vi "Router - Latency Bmk - Serial CVT FGV.vi"() -> ()   [LabVIEW 2016]
uses:
  <vilib>/Utility/error.llb/DialogType.ctl
  <vilib>/NI/Current Value Table/Type Defs/File Format.ctl
  <vilib>/NI/Current Value Table/Type Defs/Single Tag.ctl
  <vilib>/NI/Current Value Table/Type Defs/Data Types.ctl
  <vilib>/NI/Current Value Table/Type Defs/Tag Grouping set.ctl
  <vilib>/pximc/Initialize Reader Session (DBL).vi
  <vilib>/pximc/Initialize Writer Session (DBL).vi
  <vilib>/pximc/Connect (DBL).vi
  <vilib>/pximc/Read (DBL).vi
  <vilib>/pximc/Write (DBL).vi
  <vilib>/pximc/nipximc.lvlib
  <vilib>/NI/Current Value Table/Current Value Table.lvlib
panel:
  in  "Stop Button":bool
  in  "Node 2 Reader Interface":tag="PXI1Slot2" caption="interface"
  in  "Node 2 Reader Connection ID":u16=4
  in  "Node 2 Writer Interface":tag="PXI1Slot2" caption="interface"
  in  "Node 2 Writer Connection ID":u16=3
  in  "Node 1 Reader Interface":tag="PXI1Slot2" caption="interface"
  in  "Node 1 Reader Connection ID":u16=2
  in  "Node 1 Writer Interface":tag="PXI1Slot2" caption="interface"
  in  "Buffer Size":u64=250000 caption="buffer size"
  in  "Connection Timeout (s)":dbl=60.0 caption="timeout in seconds (-1)"
  in  "Node 1 Writer Connection ID":u16=1
  # "Node 1"
  # "Node 2"
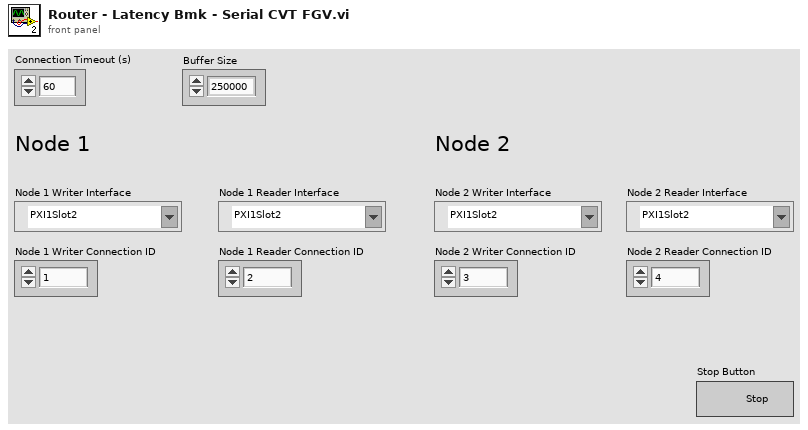
[diagram p1: front panel]
types:
  T1 = typedef "Current Value Table.lvlib/File Format.ctl" = cluster{"Tags":T2[], "Group Listings":T4[]}
  T2 = typedef "Current Value Table.lvlib/Single Tag.ctl" = cluster{"Data Type":T3, "Name":string, "Value":string, "Description":string}
  T3 = typedef "Current Value Table.lvlib/Data Types.ctl" = enum16{"Double", "Single", "I64", "I32", "I16", "I8", "U64", "U32", "U16", "U8", "String", "Boolean", "Array of U8", "Array of U16", "Array of U32", "Array of U64", "Array of I64", "Array of I32", "Array of I16", "Array of I8", "Array of Double", "Array of Single", "Array of Boolean", "Array of String"}
  T4 = typedef "Current Value Table.lvlib/Tag Grouping set.ctl" = cluster{"Group":string, "Tag Names":string[]}
  T5 = typedef "DialogType.ctl" = u16
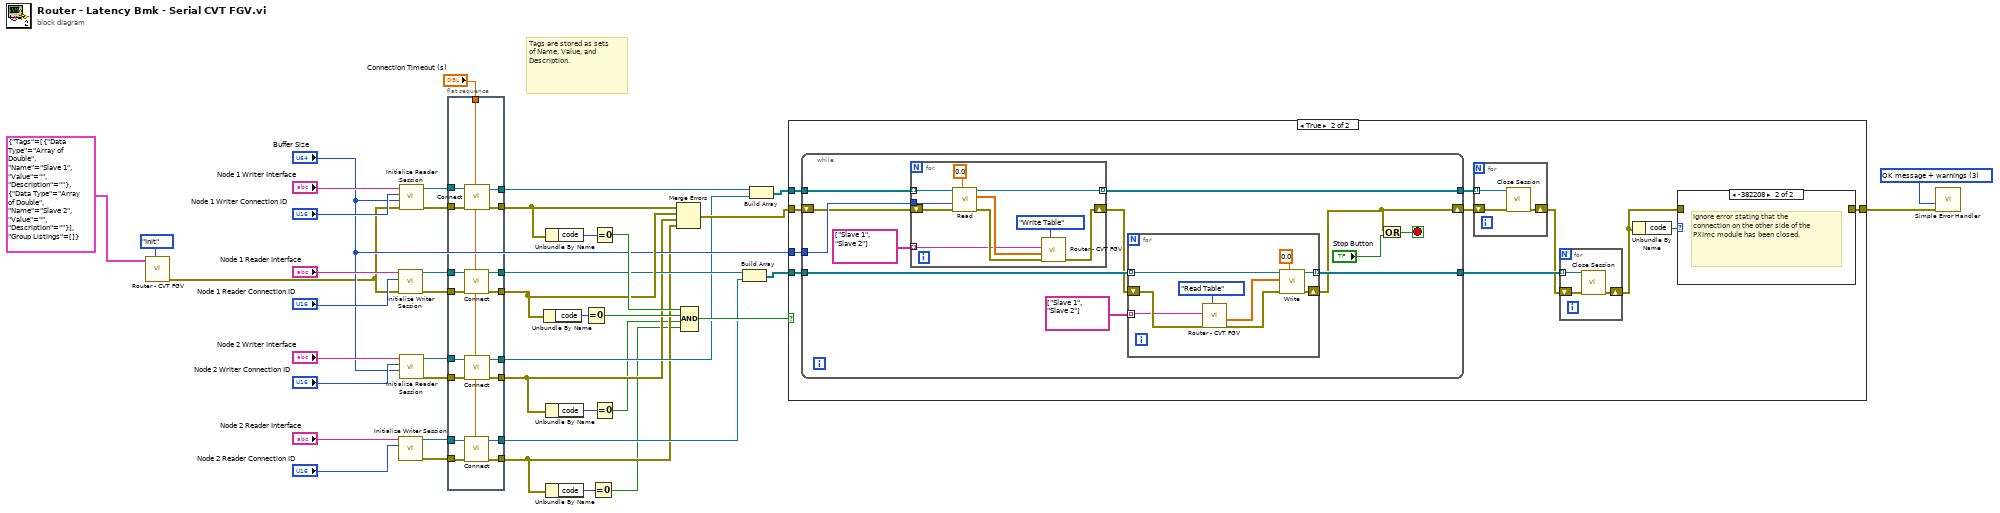
[diagram p0: block diagram]
diagram:
  w38 = T5 3 items=["no dialog", "OK message", "continue or stop message", "OK message + warnings", "continue/stop + warnings"] ("type of dialog (OK msg:1)")
  # "Tags are stored as sets of Name, Value, and Description."
  n1 = call "Router - CVT FGV.vi"("FGV Command"=enum16{"Init", "Write Table", "Read Table"}."Init", "CVT Tags to Create"=T1 {"Tags"=[{"Data Type"=enum."Array of Double", "Name"="Slave 1", "Value"="", "Description"=""}, {"Data Type"=enum."Array of Double", "Name"="Slave 2", "Value"="", "Description"=""}], "Group Listings"=[]}) -> ("error out"=w11:errorcluster)  [unwired: 8 in, 1 out]
  n2 = call-poly <vilib>:"Initialize Writer Session.vi"("error in (no error)"=w11, "connection id (1)"="Node 1 Reader Connection ID", "interface"="Node 1 Reader Interface") -> ("error out"=w36:errorcluster, "session out"=w35:refnum<k21>)  [unwired: 7 in]
  n3 = call-poly <vilib>:"Initialize Writer Session.vi"("connection id (1)"="Node 2 Reader Connection ID", "interface"="Node 2 Reader Interface") -> ("error out"=w22:errorcluster, "session out"=w23:refnum<k21>)  [unwired: 8 in]
  n4 = call-poly <vilib>:"Initialize Reader Session.vi"("error in (no error)"=w11, "buffer size"="Buffer Size", "writer's connection id (1)"="Node 1 Writer Connection ID", "interface"="Node 1 Writer Interface") -> ("error out"=w41:errorcluster, "session out"=w42:refnum<k21>)  [unwired: 6 in]
  n5 = call-poly <vilib>:"Initialize Reader Session.vi"("buffer size"="Buffer Size", "writer's connection id (1)"="Node 2 Writer Connection ID", "interface"="Node 2 Writer Interface") -> ("error out"=w18:errorcluster, "session out"=w17:refnum<k21>)  [unwired: 7 in]
  n6 = flat-sequence {
    tunnel: w42 -> [w60]
    tunnel: w41 -> [w59]
    tunnel: [w58] -> w7
    tunnel: w36 -> [w57]
    tunnel: w35 -> [w56]
    tunnel: [w55] -> w28
    tunnel: [w54] -> w27
    tunnel: "Connection Timeout (s)" -> [w44]
    tunnel: [w53] -> w9
    tunnel: [w52] -> w5
    tunnel: [w51] -> w3
    tunnel: [w50] -> w4
    tunnel: w23 -> [w49]
    tunnel: w22 -> [w48]
    tunnel: [w47] -> w6
    tunnel: w18 -> [w46]
    tunnel: w17 -> [w45]
    frame #0 {
      n7 = call-poly <vilib>:"Connect.vi"("timeout in seconds (-1)"=w44, "error in (no error)"=w57, "session in"=w56) -> ("error out"=w54:errorcluster, "session out"=w53:refnum<k21>)  [unwired: 7 in]
      n8 = call-poly <vilib>:"Connect.vi"("timeout in seconds (-1)"=w44, "error in (no error)"=w48, "session in"=w49) -> ("error out"=w51:errorcluster, "session out"=w52:refnum<k21>)  [unwired: 7 in]
      n9 = call-poly <vilib>:"Connect.vi"("timeout in seconds (-1)"=w44, "error in (no error)"=w59, "session in"=w60) -> ("error out"=w55:errorcluster, "session out"=w58:refnum<k21>)  [unwired: 7 in]
      n10 = call-poly <vilib>:"Connect.vi"("timeout in seconds (-1)"=w44, "error in (no error)"=w46, "session in"=w45) -> ("error out"=w50:errorcluster, "session out"=w47:refnum<k21>)  [unwired: 7 in]
    }
  }
  n11 = Unbundle By Name(w27) -> ("code"=w33:i32)
  n12 = Unbundle By Name(w28) -> ("code"=w39:i32)
  n13 = Unbundle By Name(w4) -> ("code"=w20:i32)
  n14 = Unbundle By Name(w3) -> ("code"=w25:i32)
  n15 = Equal To 0?(x=w33) -> (x = 0?=w30:bool)
  n16 = Equal To 0?(x=w25) -> (x = 0?=w1:bool)
  n17 = Equal To 0?(x=w39) -> (x = 0?=w31:bool)
  n18 = Equal To 0?(x=w20) -> (x = 0?=w2:bool)
  n19 = Merge Errors(w28, w27, w4, w3) -> (w29:errorcluster)
  n20 = Compound Arithmetic op=AND(w31, w30, w2, w1) -> (w32:bool)
  n21 = Build Array(w9, w5) -> (w10:refnum<k21>[])
  n22 = Build Array(w7, w6) -> (w8:refnum<k21>[])
  n23 = case shown="True" w32 {
    tunnel: w29 -> [w61 w72]
    tunnel: w8 -> [_ w71]
    tunnel: [w61 w69] -> w15
    tunnel: "Buffer Size" -> [_ w66]
    tunnel: w10 -> [_ w65]
    frame False {
      # "The connection was not successful for some reason."
    }
    frame True {
      n24 = while {
        tunnel: w71 -> [w90]
        tunnel: [w89] -> w70
        shift-right: [w81] -> w67
        shift-left: w72 -> [w84]
        tunnel: w66 -> [w88]
        tunnel: w65 -> [w87]
        tunnel: [w86] -> w64
        stop <- w85 stop-if-true
        n25 = for {
          tunnel: w88 -> [w98]
          shift-right: [w92] -> w82
          shift-left: w84 -> [w94]
          tunnel: string[] ["Slave 1", "Slave 2"] -> [w91] mode=indexing
          tunnel: w90 -> [w100] mode=indexing
          tunnel: [w99] -> w89 mode=indexing
          n26 = call-poly <vilib>:"Read.vi"("timeout in seconds (5)"=0.0, "error in (no error)"=w94, "number of elements"=w98, "session in"=w100) -> ("error out"=w93:errorcluster, "data"=w95:dbl[], "session out"=w99:refnum<k21>)  [unwired: 5 in]
          n27 = call "Router - CVT FGV.vi"("FGV Command"=enum16{"Init", "Write Table", "Read Table"}."Write Table", "error in (no error)"=w93, "Tag Array Write"=w95, "Tag Name"=w91) -> ("error out"=w92:errorcluster)  [unwired: 6 in, 1 out]
        }
        n28 = for {
          tunnel: w87 -> [w109] mode=indexing
          tunnel: [w108] -> w86 mode=indexing
          shift-right: [w107] -> w81
          shift-left: w82 -> [w103]
          tunnel: string[] ["Slave 1", "Slave 2"] -> [w101] mode=indexing
          n29 = call "Router - CVT FGV.vi"("FGV Command"=enum16{"Init", "Write Table", "Read Table"}."Read Table", "error in (no error)"=w103, "Tag Name"=w101) -> ("error out"=w102:errorcluster, "Tag Array Read"=w104:dbl[])  [unwired: 7 in]
          n30 = call-poly <vilib>:"Write.vi"("timeout in seconds (5)"=0.0, "error in (no error)"=w102, "data"=w104, "session in"=w109) -> ("error out"=w107:errorcluster, "session out"=w108:refnum<k21>)  [unwired: 5 in, 1 out]
        }
        n31 = Or(x=w81, y="Stop Button") -> (x .or. y?=w85:bool)
      }
      n32 = for {
        tunnel: w70 -> [w78] mode=indexing
        shift-right: [w76] -> w63
        shift-left: w67 -> [w77]
        n33 = call <vilib>:"Close Session.vi"("error in (no error)"=w77, "session in"=w78) -> ("error out"=w76:errorcluster)  [unwired: 9 in]
      }
      n34 = for {
        tunnel: w64 -> [w75] mode=indexing
        shift-right: [w73] -> w62
        shift-left: w63 -> [w74]
        n35 = call <vilib>:"Close Session.vi"("error in (no error)"=w74, "session in"=w75) -> ("error out"=w73:errorcluster)  [unwired: 9 in]
      }
      n36 = Unbundle By Name(w62) -> ("code"=w68:i32)
      n37 = case shown="-382208" w68 {
        tunnel: w62 -> [w110 _]
        tunnel: [w110 _] -> w69
        frame 0, Default {
        }
        frame -382208 {
          # "Ignore error stating that the connection on the other side of the PXImc module has been closed."
        }
      }
    }
  }
  n38 = call <vilib>:"Simple Error Handler.vi"("type of dialog (OK msg:1)"=w38, "error in (no error)"=w15) -> ()  [unwired: 3 in, 5 out]
